vi "Init.vi"(10 "Init Data":T2, 11 "Tasks in":refnum<class "Tasks.lvclass">) -> (3 "Tasks out":refnum<class "Tasks.lvclass">)   [LabVIEW 2012, in "Tasks.lvclass"]
uses:
  Tasks.lvclass
  Type Defs/Mode Select.ctl
  Tasks.lvclass/Tasks.ctl
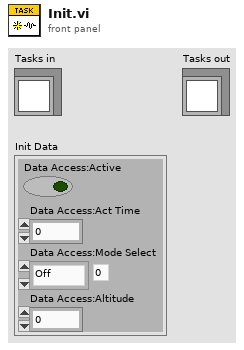
[diagram p1: front panel]
types:
  T1 = typedef "Mode Select.ctl" = enum8{"Off", "Stby", "Hold", "Run"}
  T2 = cluster{"Data Access:Active":bool, "Data Access:Act Time":sgl, "Data Access:Mode Select":T1, "Data Access:Altitude":dbl}
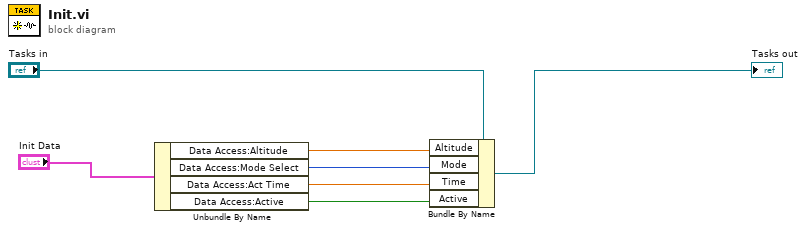
[diagram p0: block diagram]
diagram:
  n1 = Unbundle By Name("Init Data") -> ("Data Access:Altitude"=w4:dbl, "Data Access:Mode Select"=w3:T1, "Data Access:Act Time"=w2:sgl, "Data Access:Active"=w1:bool)
  n2 = Bundle By Name(cluster="Tasks in", "Altitude"=w4, "Mode"=w3, "Time"=w2, "Active"=w1) -> (→"Tasks out":refnum<class "Tasks.lvclass">)
